vi "Conveyor and Shooter SS Outputs.vi"(11 "Conveyor and Shooter Actuator Values In":T3) -> (0 "error out":T1)   [LabVIEW 2016]
uses:
  Conveyor and Shooter Actuator Out.ctl
  Conveyor and Shooter Errors.ctl
  <vilib>/Rock Robotics/WPI/ThirdParty/CanMotor/TalonSRX/WPI_CANTalonSRX_APIControlMode.ctl
  Global Variables/Refnum Names.vi
panel:
  out "Current":dbl
  out "Waveform Chart":T2(graph)
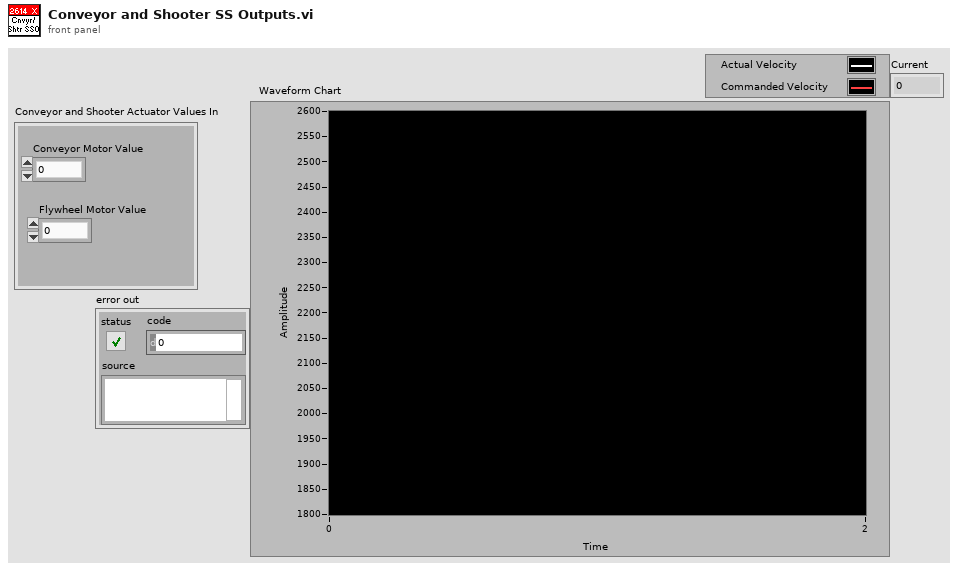
[diagram p1: front panel]
types:
  T1 = typedef "Conveyor and Shooter Errors.ctl" = errorcluster
  T2 = cluster{"Sensor Velocity":dbl, "Flywheel Motor Value":dbl}
  T3 = typedef "Conveyor and Shooter Actuator Out.ctl" = cluster{"Conveyor Motor Value":dbl, "Flywheel Motor Value":dbl}
  T4 = typedef "WPI_CANTalonSRX_APIControlMode.ctl" = enum8{"Percent VBus", "Speed", "Position", "Slave", "Unchanged / Invalid", "Voltage Compensation", "Current", "Motion Profile", "Motion Magic"}
  T5 = typedef "WPI_MotorControlDeviceRef.ctl" = cluster{"DeviceStatus":errorcluster, "Type":T6, "PWM":cluster{"PWM Channel":T7, "DeadBand":T8}, "CAN":cluster{"Device Number":u8, "SetOutput VI Ref":variant, "GetOutput VI Ref":variant, "Enable VI Ref":variant, "Disable VI Ref":variant, "Data":variant}, "Invert":bool}
  T6 = typedef "WPI_MotorControlType.ctl" = enum16{"PWM", "CAN"}
  T7 = typedef "FPGA_DIOPWMChannel.ctl" = enum8{"PWM 0", "PWM 1", "PWM 2", "PWM 3", "PWM 4", "PWM 5", "PWM 6", "PWM 7", "PWM 8", "PWM 9", "PWM MXP 0", "PWM MXP 1", "PWM MXP 2", "PWM MXP 3", "PWM MXP 4", "PWM MXP 5", "PWM MXP 6", "PWM MXP 7", "PWM MXP 8", "PWM MXP 9", "Invalid"}
  T8 = typedef "WPI_PWMDeadband.ctl" = cluster{"Name":string, "maxPositivePwm":i32, "minPositivePwm":i32, "centerPwm":i32, "maxNegativePwm":i32, "minNegativePwm":i32, "angularRange":u16}
  T9 = typedef "WPI_CANTalonSRX_GlobalStatus.ctl" = cluster{"Applied Throttle":dbl, "Module Enabled":bool, "CAN Error":errorcluster, "Closed Loop Error":dbl, "Forward Limit Switch Closed":bool, "Reverse Limit Switch Closed":bool, "Sensor Position":dbl, "Sensor Velocity":dbl, "Current":dbl, "Sticky Fault - Over Temp":bool, "Sticky Fault - Under Voltage":bool, "Sticky Fault - Forward Limit":bool, "Sticky Fault - Reverse Limit":bool, "Sticky Fault - Forward Soft Limit":bool, "Sticky Fault - Reverse Soft Limit":bool, "Brake is Enabled":bool, "Encoder Position":dbl, "Encoder Velocity":dbl, "Encoder Index Count":dbl, "Encoder A Pin State":bool, "Encoder B Pin State":bool, "Encoder Index Pin State":bool, "Analog In":dbl, "Analog In Velocity":dbl, "Temperature (C)":dbl, "Battery Voltage":dbl, "Control 5 Is Supported":bool, "Current Profile Slot Select":dbl, "Pos Div 8":bool, "Vel Div 4":bool, "Pulse Width Position":i32, "Pulse Width Velocity":i32, "Pulse Width Rise To Rise (us)":i32, "Pulse Width Rise To Fall (us)":i32, "Mot Prof Active Is Under Run":bool, "Mot Prof Active Has Under Run":bool, "Mot Prof Active Is Last":bool, "Mot Prof Active Velocity Only":bool, "Mot Prof Active Is Valid":bool, "Mot Prof Buffer Is Full":bool, "Mot Prof Active Profile Slot Select":i32, "Mot Prof NextID":i32, "Mot Prof Count":i32, "Mot Prof Active Velocity":dbl, "Mot Prof Active Position":dbl, "Mot Prof Output Enable":i32, "UsageFrame":u32, "Motion Magic Active Trajectory":cluster{"Velocity":dbl, "Position":dbl}}
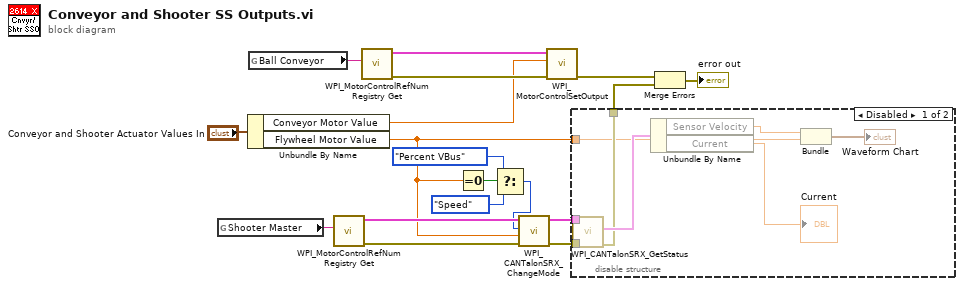
[diagram p0: block diagram]
diagram:
  n1 = global read "Refnum Names.vi" "Shooter Master"() -> (w16:string)
  n2 = Unbundle By Name("Conveyor and Shooter Actuator Values In") -> ("Conveyor Motor Value"=w6:dbl, "Flywheel Motor Value"=w5:dbl)
  n3 = global read "Refnum Names.vi" "Ball Conveyor"() -> (w14:string)
  n4 = call <vilib>:"WPI_MotorControlRefNum Registry Get.vi"("refnum name"=w16) -> ("error out"=w11:errorcluster, "MotorControlDevRef"=w17:T5)  [unwired: 9 in]
  n5 = call <vilib>:"WPI_MotorControlRefNum Registry Get.vi"("refnum name"=w14) -> ("error out"=w10:errorcluster, "MotorControlDevRef"=w15:T5)  [unwired: 9 in]
  n6 = Equal To 0?(x=w5) -> (x = 0?=w4:bool)
  n7 = Select(t=WPI_CANTalonSRX_APIControlMode."Percent VBus" ("Control Mode"), s=w4, f=WPI_CANTalonSRX_APIControlMode."Speed" ("Control Mode")) -> (s? t:f=w2:T4)
  n8 = call <vilib>:"WPI_CANTalonSRX_ChangeMode.vi"("error in (no error)"=w11, "Output"=w5, "Control Mode"=w2, "CAN Talon SRX Ref"=w17) -> ("error out"=w12:errorcluster, "CAN Talon SRX Ref"=w13:T5)  [unwired: 6 in]
  n9 = call <vilib>:"WPI_MotorControlSetOutput.vi"("error in (no error)"=w10, "Output"=w6, "MotorControlDevRef"=w15) -> ("error out"=w8:errorcluster)  [unwired: 6 in, 2 out]
  n10 = disable-structure shown="Disabled" {
    disable-tunnel: w13 -> [w26 _]
    disable-tunnel: w12 -> [w22 _]
    disable-tunnel: [w21 _] -> w9
    disable-tunnel: w5 -> [w20 _]
    frame Disabled {
      n11 = call <vilib>:"WPI_CANTalonSRX_GetStatus.vi"("error in (no error)"=w22, "CAN Talon SRX Ref"=w26) -> ("error out"=w21:errorcluster, "Talon SRX Status"=w25:T9)  [unwired: 7 in, 1 out]
      n12 = Unbundle By Name(w25) -> ("Sensor Velocity"=w24:dbl, "Current"=→"Current":dbl)
      n13 = Bundle("Sensor Velocity"=w24, "Flywheel Motor Value"=w20) -> (→"Waveform Chart":T2)  [unwired: 1 in]
    }
    frame Enabled {
    }
  }
  n14 = Merge Errors(w8, w9) -> (→"error out":errorcluster)
